vi "PH_BackreflectionMeas.PC Write PSDB.vi"(0 "i ref in":refnum<vi>, 5 "error IO":errorcluster) -> (14 "i ref out":refnum<vi>, 19 "error out":errorcluster)   [LabVIEW 2014, in "PH_BackreflectionMeas.lvlib"]
doc: "This is the proc case which writes data to the PHELIX shot data base."
uses:
  PH_BackreflectionMeas.lvlib
  PH_Basics/PH_PSDBWriter/PH_PSDBWriter.lvlib
  PH_Basics/PH_StatusHandler/PH_StatusHandler.lvlib
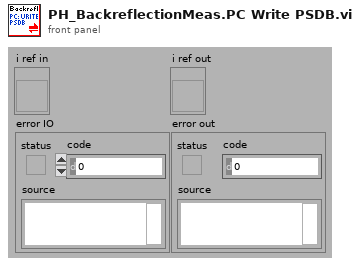
[diagram p1: front panel]
types:
  T1 = typedef "PH_PSDBWriter.lvlib/PH_PSDBWriter.String dataset.ctl" = cluster{"name":string, "data":string, "unit":string}
  T2 = typedef "PH_PSDBWriter.lvlib/PH_PSDBWriter.2D dataset.ctl" = cluster{"name":string, "data":dbl[][], "axis description":T3}
  T3 = typedef "PSDB.lvlib/PSDB_AxisDescription.ctl" = cluster{"x axis label":string, "y axis label":string, "x axis unit":string, "y axis unit":string}
  T4 = typedef "PH_PSDBWriter.lvlib/PH_PSDBWriter.PSDB Dataset.ctl" = cluster{"Version":i32, "2D data Input":T2[], "Boolean Input":T5[], "Image Input":T6[], "Numeric Input":T8[], "String Input":T1[]}
  T5 = typedef "PH_PSDBWriter.lvlib/PH_PSDBWriter.Boolean dataset.ctl" = cluster{"name":string, "data":bool, "unit":string}
  T6 = typedef "PH_PSDBWriter.lvlib/PH_PSDBWriter.Image dataset.ctl" = cluster{"name":string, "data":T7, "unit":string}
  T7 = typedef "IMAQ Image.ctl" = refnum<image>
  T8 = typedef "PH_PSDBWriter.lvlib/PH_PSDBWriter.Numeric dataset.ctl" = cluster{"name":string, "data":dbl, "unit":string}
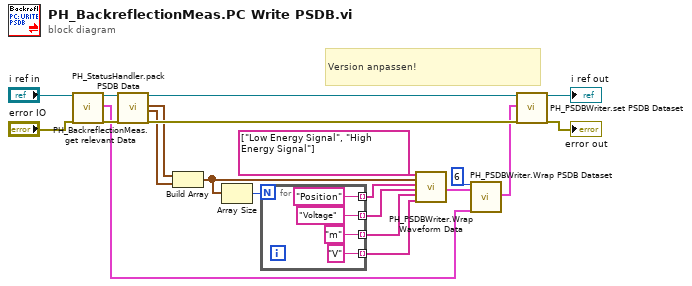
[diagram p0: block diagram]
diagram:
  # "Version anpassen!"
  n1 = call "PH_StatusHandler.pack PSDB Data.vi"("VI in"="i ref in", "error in (no error)"="error IO") -> ("VI out"=w21:refnum<vi>, "PSDB String Data Array"=w1:T1[], "error out"=w20:errorcluster)  [unwired: 15 in]
  n2 = call "PH_BackreflectionMeas.get relevant Data.vi"("i ref in"=w21, "error in"=w20) -> ("i ref out"=w13:refnum<vi>, "low Energy Waveform"=w16:waveform(dbl), "high Energy Waveform"=w15:waveform(dbl), "error out"=w19:errorcluster)  [unwired: 14 in]
  n3 = Build Array(w16, w15) -> (w7:waveform(dbl)[])
  n4 = Array Size(array=w7) -> (size(s)=w6:i32)
  n5 = for {
    N: w6 -> [_]
    tunnel: ["Position" ("x axis label")] -> w5 mode=indexing
    tunnel: ["Voltage" ("y axis label")] -> w4 mode=indexing
    tunnel: ["m" ("x axis unit")] -> w3 mode=indexing
    tunnel: ["V" ("y axis unit")] -> w2 mode=indexing
  }
  n6 = call "PH_PSDBWriter.Wrap Waveform Data.vi"("Name Array"=string[] ["Low Energy Signal", "High Energy Signal"], "Data Array"=w7, "x axis label Array"=w5, "y axis label Array"=w4, "x axis unit Array"=w3, "y axis unit Array"=w2) -> ("PSDB 2D Data Array"=w10:T2[])  [unwired: 13 in]
  n7 = call "PH_PSDBWriter.Wrap PSDB Dataset.vi"("Version"=6, "2D data Input"=w10, "String Input"=w1) -> ("PSDB Dataset"=w9:T4)  [unwired: 16 in]
  n8 = call "PH_PSDBWriter.set PSDB Dataset.vi"("VI in"=w13, "PSDB Dataset"=w9, "error in (no error)"=w19) -> ("VI out"=→"i ref out":refnum<vi>, "error out"=→"error out":errorcluster)  [unwired: 15 in]
